vi "I2C_Read_1_Byte_DAQ.vi"() -> (2 "Byte.Data.Read":u8 format="%02x")   [LabVIEW 2022 SP3]
doc: "Petrus Prins 7 June 2026"
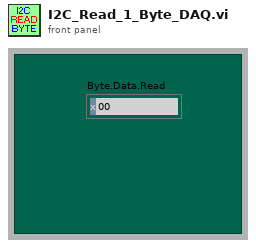
[diagram p1: front panel]
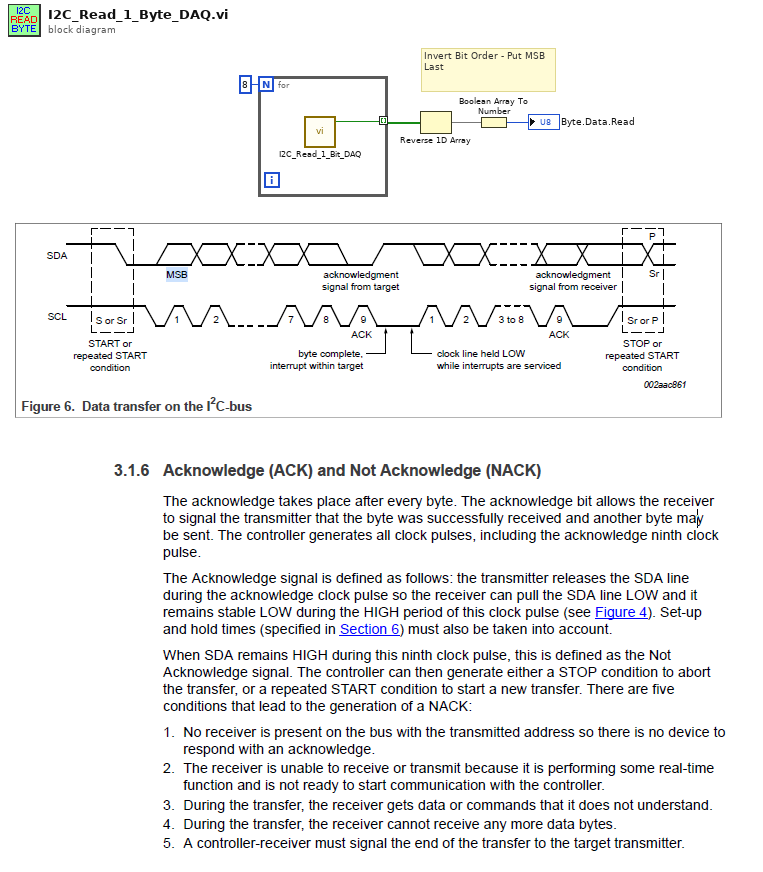
[diagram p0: block diagram]
diagram:
  # "Invert Bit Order - Put MSB Last"
  n1 = for {
    N: 8 -> [_]
    tunnel: [w5] -> w3 mode=indexing
    n2 = call "I2C_Read_1_Bit_DAQ.vi"() -> ("RX_Bit_Out"=w5:bool)  [unwired: 2 in]
  }
  n3 = Reverse 1D Array(array=w3) -> (reversed array=w2:bool[])
  n4 = Boolean Array To Number(Boolean array=w2) -> (number=→"Byte.Data.Read":u8)
